vi "multiple_peak_finder.vi"(1 "FFT in":dbl[][](array[numeric])) -> (0 "Indices":i32[](array[numeric]))   [LabVIEW 2009]
panel:
  out "Fundamental Frequency":dbl
  out "Peaks":dbl[](array[numeric])
  out "Array":i32[](array[numeric])
  in  "number of peaks":i32(slide)=4 scale=0.0..6.0
  out "Array 3":i32[](array[numeric])
  out "Array 2":bool[](array[boolean])
  in  "Threshold":dbl(slide)=0.04 scale=0.0..0.4
  out "first order derivative":dbl[](graph)
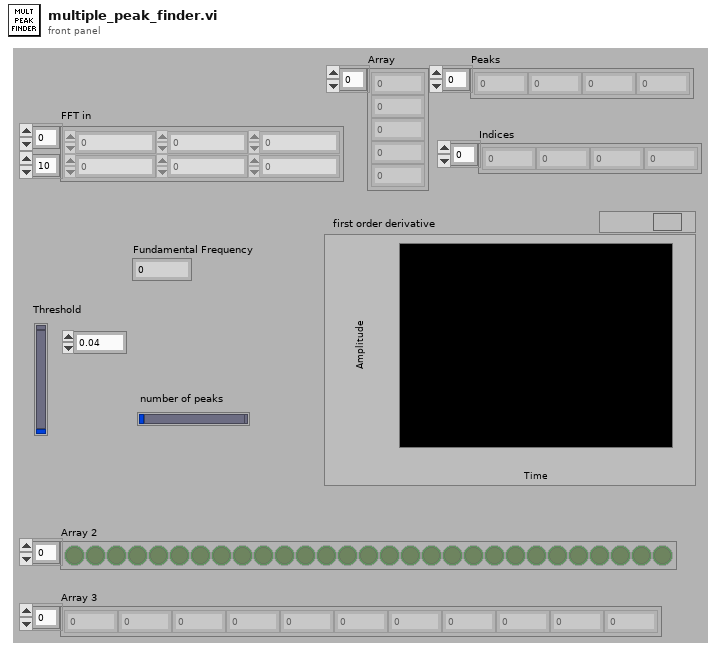
[diagram p1: front panel]
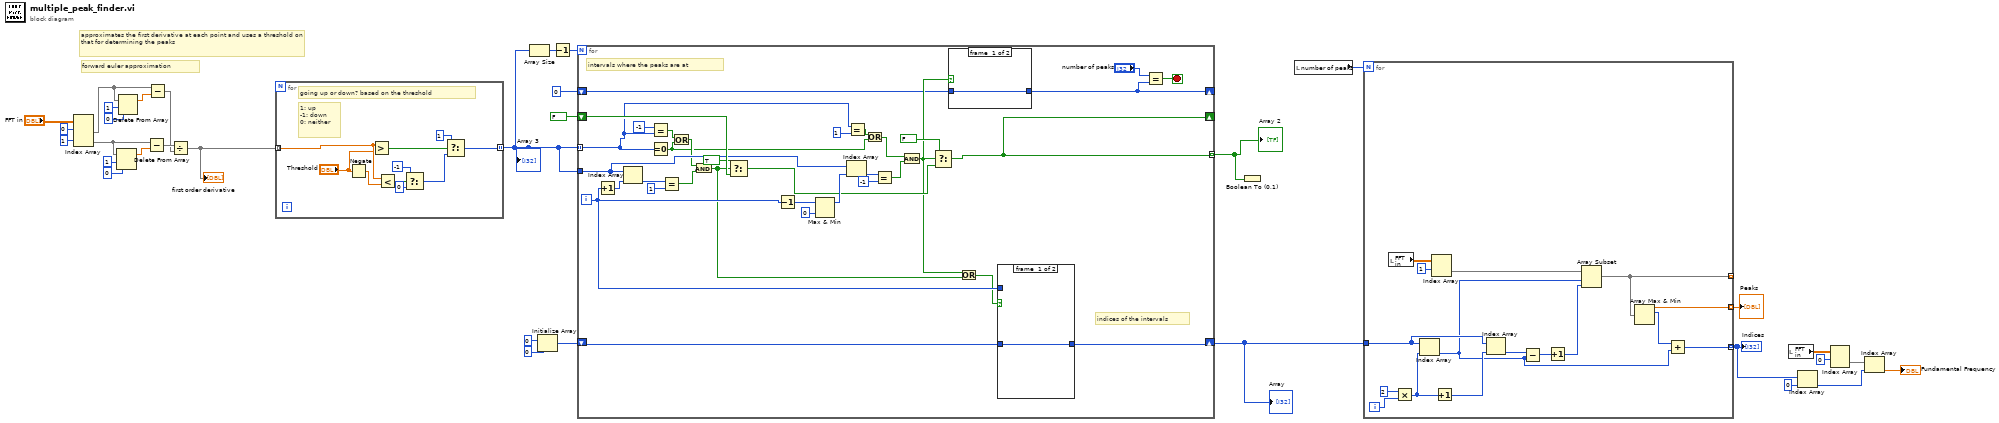
[diagram p0: block diagram]
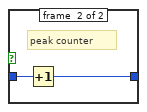
[diagram p2: hidden frame]
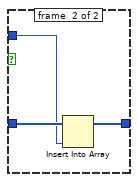
[diagram p3: hidden frame]
diagram:
  # "forward euler approximation"
  # "approximates the first derivative at each point and uses a threshold on that for determining the peaks"
  n1 = Index Array(array="FFT in", index (row) #1=0 ("index (row)"), index (row) #2=1 ("index (row)")) -> (element #1=w22:dbl[], element #2=w28:dbl[])  [unwired: 2 in]
  n2 = Delete From Array(array=w28, length=1, index=0) -> (array with subset deleted=w27:dbl[])  [unwired: 1 out]
  n3 = Delete From Array(array=w22, length=1, index=0) -> (array with subset deleted=w23:dbl[])  [unwired: 1 out]
  n4 = Subtract(x=w28, y=w27) -> (x-y=w26:dbl[])
  n5 = Subtract(x=w22, y=w23) -> (x-y=w21:dbl[])
  n6 = Divide(x=w26, y=w21) -> (x/y=w20:dbl[])
  "first order derivative" <- w20
  n7 = for {
    tunnel: w20 -> [w40] mode=indexing
    tunnel: [w35] -> w17 mode=indexing
    # "1: up\n-1: down\n0: neither"
    # "going up or down? based on the threshold"
    n8 = Negate(x="Threshold") -> (-x=w41:dbl)
    n9 = Greater?(x=w40, y="Threshold") -> (0:w43:bool)
    n10 = Less?(x=w40, y=w41) -> (x < y?=w39:bool)
    n11 = Select(t=-1, s=w39, f=0) -> (s? t:f=w36:i32)
    n12 = Select(t=1, s=w43, f=w36) -> (s? t:f=w35:i32)
  }
  "Array 3" <- w17
  n13 = Array Size(array=w17) -> (size(s)=w19:i32)
  n14 = Initialize Array(0 ("element"), 0 ("dimension size")) -> (w13:i32[])
  n15 = Decrement(x=w19) -> (x-1=w18:i32)
  n16 = for {
    N: w18 -> [_]
    tunnel: w17 -> [w48] mode=indexing
    tunnel: w17 -> [w72]
    shift-right: [w62] -> _
    shift-left: FALSE -> [w73]
    tunnel: [w62] -> w11 mode=indexing
    shift-right: [w58] -> w9
    shift-left: w13 -> [w59]
    shift-right: [w53] -> _
    shift-left: 0 -> [w55]
    i -> [w63]
    stop <- w52 stop-if-true
    # "indices of the intervals"
    # "intervals where the peaks are at"
    n17 = Increment(x=w63) -> (x+1=w77:i32)
    n18 = Index Array(array=w72, index=w77) -> (element=w76:i32)
    n19 = Equal?(x=-1, y=w48) -> (x = y?=w50:bool)
    n20 = Equal To 0?(x=w48) -> (x = 0?=w44:bool)
    n21 = Equal?(x=w76, y=1) -> (x = y?=w74:bool)
    n22 = Or(x=w50, y=w44) -> (x .or. y?=w49:bool)
    n23 = And(x=w49, y=w74) -> (x .and. y?=w57:bool)
    n24 = Select(t=TRUE, s=w57, f=w73) -> (s? t:f=w61:bool)
    n25 = Decrement(x=w63) -> (x-1=w69:i32)
    n26 = Max & Min(x=w69, y=0) -> (max(x,y)=w70:i32)  [unwired: 1 out]
    n27 = Index Array(array=w72, index=w70) -> (element=w68:i32)
    n28 = Equal?(x=w48, y=1) -> (x = y?=w46:bool)
    n29 = Or(x=w46, y=w44) -> (x .or. y?=w45:bool)
    n30 = Equal?(x=w68, y=-1) -> (x = y?=w66:bool)
    n31 = And(x=w45, y=w66) -> (x .and. y?=w56:bool)
    n32 = Select(t=FALSE, s=w56, f=w61) -> (s? t:f=w62:bool)
    n33 = case shown="True" w56 {
      tunnel: w55 -> [w78 w80]
      tunnel: [w78 w79] -> w53
      frame #0 {
      }
      frame #1 {
        # "peak counter"
        n34 = Increment(x=w80) -> (x+1=w79:i32)
      }
    }
    n35 = Or(x=w56, y=w57) -> (x .or. y?=w60:bool)
    n36 = case shown="True" w60 {
      tunnel: w63 -> [_ w83]
      tunnel: w59 -> [w81 w84]
      tunnel: [w81 w82] -> w58
      frame #0 {
      }
      frame #1 {
        n37 = Insert Into Array(array=w84, new element=w83) -> (w82:i32[])  [unwired: 1 in]
      }
    }
    n38 = Equal?(x="number of peaks", y=w53) -> (x = y?=w52:bool)
  }
  "Array 2" <- w11
  "Array" <- w9
  n39 = Boolean To (0,1)(Boolean=w11) -> ()  [unwired: 1 out]
  n40 = local read "number of peaks"() -> (w10:i32)
  n41 = for {
    N: w10 -> [_]
    tunnel: w9 -> [w97]
    tunnel: [w89] -> _ mode=indexing
    tunnel: [w88] -> w8 mode=indexing
    tunnel: [w85] -> w5 mode=indexing
    i -> [w100]
    n42 = local read "FFT in"() -> (w95:dbl[][])
    n43 = Multiply(x=2, y=w100) -> (x*y=w98:i32)
    n44 = Index Array(array=w97, index=w98) -> (element=w86:i32)
    n45 = Index Array(array=w95, index (row)=1 ("disabled index (col)")) -> (element=w93:dbl[])  [unwired: 1 in]
    n46 = Increment(x=w98) -> (x+1=w96:i32)
    n47 = Index Array(array=w97, index=w96) -> (element=w92:i32)
    n48 = Subtract(x=w92, y=w86) -> (x-y=w91:i32)
    n49 = Increment(x=w91) -> (x+1=w90:i32)
    n50 = Array Subset(array=w93, index=w86, length=w90) -> (w89:dbl[])
    n51 = Array Max & Min(array=w89) -> (max value=w88:dbl, max index (indices)=w87:i32)  [unwired: 2 out]
    n52 = Add(x=w87, y=w86) -> (x+y=w85:i32)
  }
  "Peaks" <- w8
  "Indices" <- w5
  n53 = local read "FFT in"() -> (w7:dbl[][])
  n54 = Index Array(array=w5, index=0) -> (element=w2:i32)
  n55 = Index Array(array=w7, index (row)=0) -> (element=w3:dbl[])  [unwired: 1 in]
  n56 = Index Array(array=w3, index=w2) -> (element=→"Fundamental Frequency":dbl)
